vi "Clear UIMsg Callbacks.vi"(8 "error in (no error)":errorcluster, 11 "Execution in":refnum<class "Execution.lvclass">) -> (0 "error out":errorcluster, 3 "Execution out":refnum<class "Execution.lvclass">)   [LabVIEW 2020, in "TSnax.lvlib" / "Execution.lvclass"]
uses:
  Execution.lvclass
  Execution.lvclass/Execution.ctl
  UIMessage Callback.vi
  Engine/Engine.lvclass
  UIMessage/UIMessage.lvclass
  C:/dev/illuminated-g/tsnax/TSnax/PropertyObject/PropertyObject.lvclass
  C:/dev/illuminated-g/tsnax/TSnax/UIMessage/UIMessage.lvclass
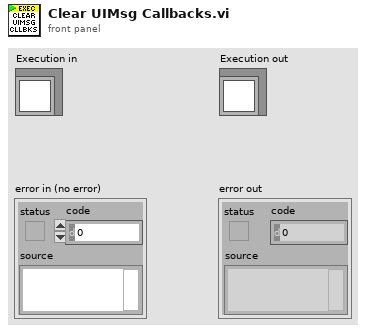
[diagram p1: front panel]
types:
  T1 = typedef "TSnax.lvlib/UIMsg.ctl" = enum16{"Unknown", "BreakOnUserRequest", "BreakOnBreakpoint", "BreakOnRunTimeError", "Trace", "TerminatingExecution", "AbortingExecution", "KillingExecutionThreads", "EndExecution", "ShutDownComplete", "StartExecution", "ProgressPercent", "ProgressText", "StartInteractiveExecution", "EndInteractiveExecution", "TerminatingInteractiveExecution", "TerminationCancelled", "ResumeFromBreak", "StartFileExecution", "EndFileExecution", "ShutDownCancelled", "LocalizationSettingChanged", "OpenWindows", "TileWindows", "CascadeWindows", "ReportChanged", "CloseWindows", "RefreshWindows", "ClientFileChanged", "DisplayReport", "ModelState_Initializing", "ModelState_Waiting", "ModelState_Identified", "ModelState_BeginTesting", "ModelState_TestingComplete", "ModelState_PostProcessingComplete", "ModelState_EnabledStateSet", "ReportLocationChanged", "GotoLocation", "PushUndoItem", "OutputMessages", "TypePaletteFileListChanged", "NonTerminatingThreadsArePreventingTermination", "ModelState_PostProcessing", "ReportCollectionChanged", "RuntimeError"}
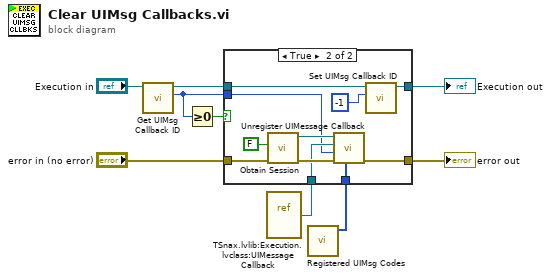
[diagram p0: block diagram]
diagram:
  n1 = call "Get UIMsg Callback ID.vi"("Execution in"="Execution in") -> ("UIMsg Callback ID"=w2:i32, "Execution out"=w4:refnum<class "Execution.lvclass">)  [unwired: 8 in, 1 out]
  n2 = Greater Or Equal To 0?(x=w2) -> (x >= 0?=w1:bool)
  n3 = vi-ref "TSnax.lvlib:Execution.lvclass:UIMessage Callback.vi"() -> (w8:refnum<vi>)
  n4 = call "Registered UIMsg Codes.vi"() -> ("UIMessage Codes"=w9:T1[])  [unwired: 11 in]
  n5 = case shown="True" w1 {
    tunnel: w9 -> [_ w20]
    tunnel: w8 -> [_ w18]
    tunnel: "error in (no error)" -> [w10 w17]
    tunnel: [w10 w16] -> w6
    tunnel: w4 -> [w11 w15]
    tunnel: [w11 w14] -> w3
    tunnel: w2 -> [_ w12]
    frame False {
    }
    frame True {
      n6 = call "Obtain Session.vi"("error in (no error)"=w17, "Create if needed? (T)"=FALSE) -> ("error out"=w19:errorcluster, "Engine out"=w21:refnum<class "Engine.lvclass">)  [unwired: 8 in]
      n7 = call "Unregister UIMessage Callback.vi"("UIMessage IDs"=w20, "error in (no error)"=w19, "Callback ID"=w12, "Callback"=w18, "Engine in"=w21) -> ("error out"=w16:errorcluster)  [unwired: 5 in, 1 out]
      n8 = call "Set UIMsg Callback ID.vi"("UIMsg Callback ID"=-1, "Execution in"=w15) -> ("Execution out"=w14:refnum<class "Execution.lvclass">)  [unwired: 8 in, 1 out]
    }
  }
  "error out" <- w6
  "Execution out" <- w3
